vi "DFD Halfband Design.vi"(4 "filtering mode":T1=2 items=["No Rate Change", "Interpolation", "Decimation"], 5 "method":u16(ring)=3 items=["Kaiser Window", "Dolph-Chebyshev Window", "Equi-Ripple", "Positive Equi-Ripple", "Max Flat"], 6 "fs in [Hz]":dbl=1.0 format="%.2f", 7 "filter type":enum16{"Lowpass", "Highpass"}(ring), 8 "error in (no error)":errorcluster, 9 "stopband attenuation [dB]":dbl=40.0 format="%.2f", 10 "roll off":dbl=0.2, 11 "order":i32=-1) -> (0 "error out":errorcluster, 2 "order out":i32, 3 "multirate filter out":T2={"mMRate_Structure"=enum."IIR", "mMRate_Mode"=0, "mMRate_Factor"=-1, "mMRate_FIRParams"={"mMRate_FIR_H"=[], "mMRate_FIR_IsNyquist?"=FALSE, "mMRate_FIR_IsSymmetric?"=FALSE}, "mMRate_CICParams"={"mMRate_CIC_#Stage"=0, "mMRate_CIC_Lag"=0, "mMRate_CIC_Type"=enum."Lowpass"}, "mMRate_Order"=0, "mMRate_Version"="2.0", "mMRate_Comments"="", "mMRate_RationalFactor"={"mMRate_L"=-1, "mMRate_M"=-1}, "mMRate_Fs"=1.0, "mMRate_Quantized?"=FALSE, "mMRate_QFilterGain"=1.0, "mMRate_CoefWl"=16, "mMRate_Scaling"={"mMRate_ScaleByPowerOf2?"=FALSE, "mMRate_ScaleType"=enum."No Norm"}, "mMRate_InputWl"=16, "mMRate_OutputWl"=16, "mMRate_OutputMode"=enum."Truncation", "mMRate_MultMode"=enum."Truncated", "mMRate_BitPruning"=FALSE, "mMRate_GainWl"=16, "mMRate_OutputFwl"=0, "mMRate_SumIwl"=0, "mMRate_InputIwl "=16, "mMRate_SumWl"=32, "mMRate_CoefIwl"=0} {"mMRate_SumWl" min=1 max=32 step=1; "mMRate_InputIwl" min=1 max=32 step=1; "mMRate_GainWl" min=1 max=32 step=1; "mMRate_OutputWl" min=1 max=32 step=1; "mMRate_InputWl" min=1 max=32 step=1; "mMRate_CoefWl" min=1 max=32 step=1; "mMRate_Mode" items=["Default"=-1, "No Rate Change"=0, "Interpolation"=1, "Decimation"=2, "Interpolated"=3, "Rational"=4]})   [LabVIEW 2017, in "NI_DigFilterLicensed.lvlib"]
doc: "Creates a halfband filter with an automatic order estimation."
uses:
  <vilib>/addons/Digital Filter Design/NI_DigFilterLicensed.lvlib
  <vilib>/addons/Digital Filter Design/_Objects.llb/DFD Multirate Filter Obj.ctl
  <vilib>/addons/Digital Filter Design/_Objects.llb/DFD Multirate Mode.ctl
  <vilib>/addons/Digital Filter Design/_Objects.llb/DFD Coef Norm Type.ctl
  <vilib>/addons/Digital Filter Design/_Objects.llb/DFD Round-off Mode.ctl
  <vilib>/addons/Digital Filter Design/_Objects.llb/DFD FXP MRate Multiply Mode.ctl
  <vilib>/addons/Digital Filter Design/_Objects.llb/DFD Multirate Filtering Mode.ctl
  <vilib>/addons/Digital Filter Design/NI_DigFilter_Process.lvlib
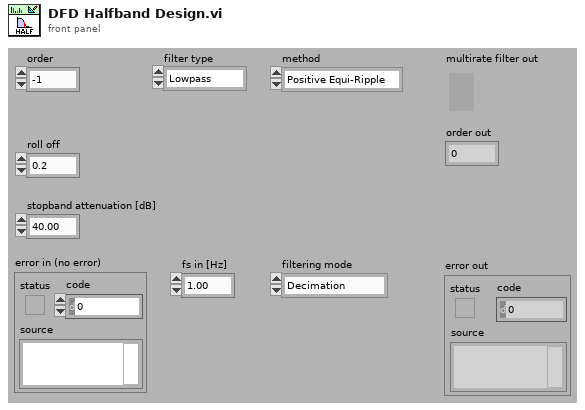
[diagram p1: front panel]
types:
  T1 = typedef "NI_DigFilterLicensed.lvlib/DFD Multirate Filtering Mode.ctl" = u16
  T2 = typedef "NI_DigFilterLicensed.lvlib/DFD Multirate Filter Obj.ctl" = cluster{"mMRate_Structure":enum16{"CIC", "FIR", "IIR", "Lattice"}, "mMRate_Mode":T3, "mMRate_Factor":i32, "mMRate_FIRParams":cluster{"mMRate_FIR_H":dbl[], "mMRate_FIR_IsNyquist?":bool, "mMRate_FIR_IsSymmetric?":bool}, "mMRate_CICParams":cluster{"mMRate_CIC_#Stage":i32, "mMRate_CIC_Lag":i32, "mMRate_CIC_Type":enum16{"Lowpass", "Highpass"}}, "mMRate_Order":i32, "mMRate_Version":string, "mMRate_Comments":string, "mMRate_RationalFactor":cluster{"mMRate_L":i32, "mMRate_M":i32}, "mMRate_Fs":dbl, "mMRate_Quantized?":bool, "mMRate_QFilterGain":dbl, "mMRate_CoefWl":i16, "mMRate_Scaling":cluster{"mMRate_ScaleByPowerOf2?":bool, "mMRate_ScaleType":T4}, "mMRate_InputWl":i16, "mMRate_OutputWl":i16, "mMRate_OutputMode":T5, "mMRate_MultMode":T6, "mMRate_BitPruning":bool, "mMRate_GainWl":i16, "mMRate_OutputFwl":i16, "mMRate_SumIwl":i16, "mMRate_InputIwl ":i16, "mMRate_SumWl":i16, "mMRate_CoefIwl":i16}
  T3 = typedef "NI_DigFilterLicensed.lvlib/DFD Multirate Mode.ctl" = i16
  T4 = typedef "NI_DigFilterLicensed.lvlib/DFD Coef Norm Type.ctl" = enum16{"No Norm", "Time Domain 1-Norm", "Time Domain 2-Norm", "Time Domain Inf-Norm"}
  T5 = typedef "NI_DigFilterLicensed.lvlib/DFD Round-off Mode.ctl" = enum16{"Nearest", "Truncation"}
  T6 = typedef "NI_DigFilterLicensed.lvlib/DFD FXP MRate Multiply Mode.ctl" = enum16{"Truncated", "Full"}
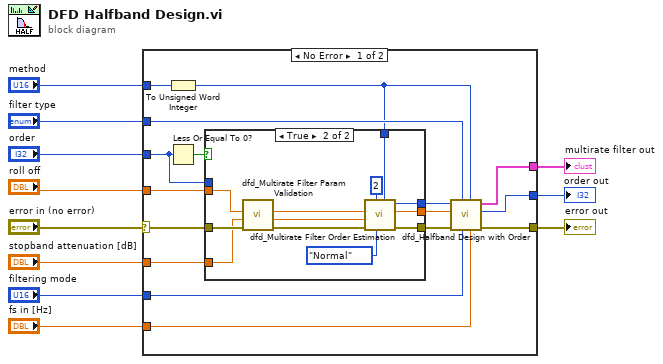
[diagram p0: block diagram]
diagram:
  n1 = case shown="No Error" "error in (no error)" {
    selector: "error in (no error)" -> [w13 w43]
    tunnel: "filter type" -> [w27 _]
    tunnel: [w26 w43] -> w10
    tunnel: [w25 _] -> w9
    tunnel: "method" -> [w24 _]
    tunnel: "roll off" -> [w23 _]
    tunnel: "filtering mode" -> [w22 _]
    tunnel: [w21 _] -> w5
    tunnel: "stopband attenuation [dB]" -> [w17 _]
    tunnel: "order" -> [w15 _]
    tunnel: "fs in [Hz]" -> [w12 _]
    frame No Error {
      n2 = To Unsigned Word Integer(number=w24) -> (unsigned 16bit integer=w14:u16)
      n3 = Less Or Equal To 0?(x=w15) -> (x <= 0?=w16:bool)
      n4 = case shown="True" w16 {
        tunnel: w14 -> [_ w42]
        tunnel: w23 -> [w30 w41]
        tunnel: w13 -> [w29 w40]
        tunnel: [w29 w39] -> w20
        tunnel: [w28 w38] -> w19
        tunnel: [w30 w35] -> w18
        tunnel: w17 -> [_ w33]
        tunnel: w15 -> [w28 _]
        frame False {
        }
        frame True {
          n5 = call <vilib>:"dfd_Multirate Filter Param Validation.vi"("error in (no error)"=w40, "A Stop [dB]"=w33, "roll off"=w41) -> ("error out"=w37:errorcluster, "dup A Stop [dB]"=w32:dbl, "dup roll off"=w36:dbl)  [unwired: 5 in, 1 out]
          n6 = call <vilib>:"dfd_Multirate Filter Order Estimation.vi"("method"=w42, "band option"=enum16{"Normal", "Nyquist", "Alias free"}."Normal", "multirate factor"=2 ("#band"), "error in (no error)"=w37, "A Stop [dB]"=w32, "roll off"=w36) -> ("error out"=w39:errorcluster, "dup roll off"=w35:dbl, "new order"=w38:i32)  [unwired: 2 in, 1 out]
        }
      }
      n7 = call <vilib>:"dfd_Halfband Design with Order.vi"("fs in [Hz]"=w12, "method"=w14, "filtering mode"=w22, "filter type"=w27, "error in (no error)"=w20, "roll off"=w18, "order"=w19) -> ("error out"=w26:errorcluster, "order out"=w21:i32, "multirate filter out"=w25:T2)  [unwired: 2 out]
    }
    frame Error {
    }
  }
  "error out" <- w10
  "multirate filter out" <- w9
  "order out" <- w5
